vi "cell_temp_values.vi"(2 "Temp In":dbl[](array[numeric]), 3 "lower limit":i32, 4 "Temp":dbl, 5 "Temp Id":i32, 6 "upper limit":i32) -> (0 "Temp Out":dbl[](array[numeric]))   [LabVIEW 2017]
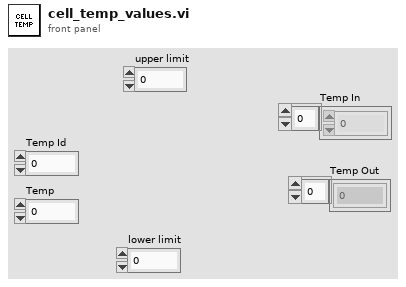
[diagram p1: front panel]
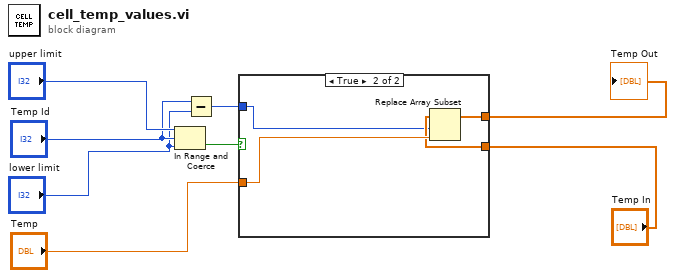
[diagram p0: block diagram]
diagram:
  n1 = In Range and Coerce(upper limit="upper limit", x="Temp Id", lower limit="lower limit") -> (In Range?=w8:bool)  [unwired: 1 out]
  n2 = Subtract(x="Temp Id", y="lower limit") -> (x-y=w7:i32)
  n3 = case shown="True" w8 {
    tunnel: [w9 w12] -> w2
    tunnel: "Temp" -> [_ w13]
    tunnel: w7 -> [_ w10]
    tunnel: "Temp In" -> [w9 w11]
    frame False {
    }
    frame True {
      n4 = Replace Array Subset(array=w11, new element=w13, index=w10) -> (w12:dbl[])
    }
  }
  "Temp Out" <- w2
